vi "Set Control Values v2.vi"(6 "class names":string[](array[string]), 8 "error in":errorcluster, 9 "values":dbl[](array[numeric]), 11 "refnums in":refnum<vi>[](array[refnum])) -> (0 "error out":errorcluster, 3 "refnums out":refnum<vi>[](array[refnum]))   [LabVIEW 2020]
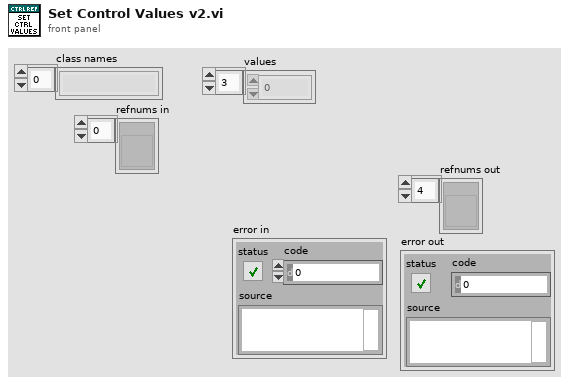
[diagram p1: front panel]
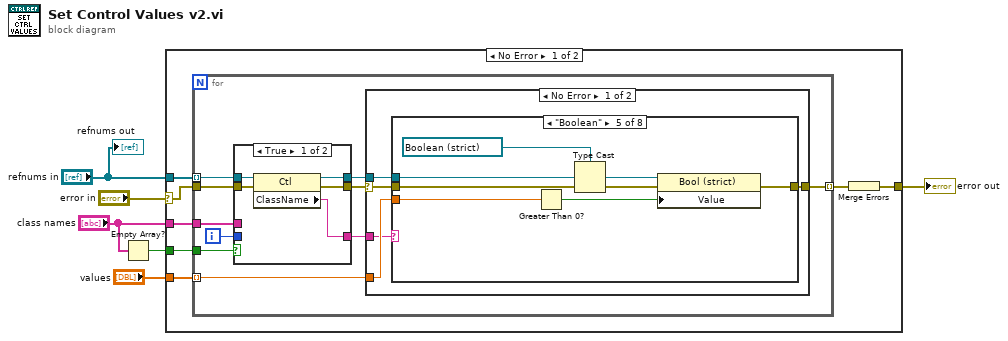
[diagram p0: block diagram]
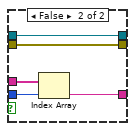
[diagram p2: hidden frame]
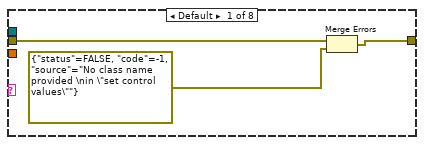
[diagram p3: hidden frame]
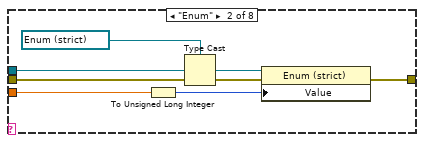
[diagram p4: hidden frame]
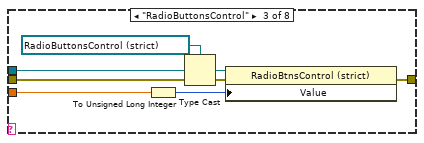
[diagram p5: hidden frame]
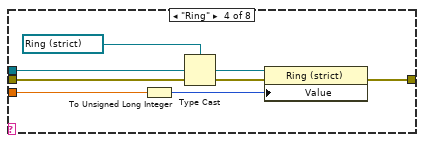
[diagram p6: hidden frame]
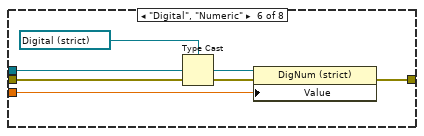
[diagram p7: hidden frame]
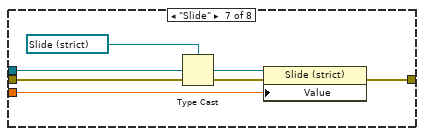
[diagram p8: hidden frame]
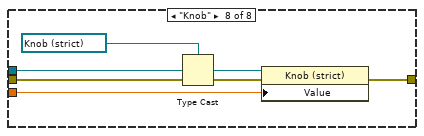
[diagram p9: hidden frame]
diagram:
  n1 = Empty Array?(array="class names") -> (empty?=w3:bool)
  n2 = case shown="No Error" "error in" {
    selector: "error in" -> [w10 w89]
    tunnel: "refnums in" -> [w12 _]
    tunnel: [w11 w89] -> w5
    tunnel: w3 -> [w9 _]
    tunnel: "class names" -> [w8 _]
    tunnel: "values" -> [w7 _]
    frame No Error {
      n3 = for {
        tunnel: w12 -> [w23] mode=indexing
        tunnel: [w21] -> w13 mode=indexing
        tunnel: w10 -> [w19]
        tunnel: w9 -> [w18]
        tunnel: w8 -> [w16]
        tunnel: w7 -> [w14] mode=indexing
        i -> [w15]
        n4 = case shown="True" w18 {
          tunnel: w23 -> [w28 w33]
          tunnel: [w27 w33] -> w22
          tunnel: [w26 w32] -> w20
          tunnel: w19 -> [w25 w32]
          tunnel: [w24 w30] -> w17
          tunnel: w16 -> [_ w31]
          tunnel: w15 -> [_ w29]
          frame True {
            n5 = property class="Ctl"(reference=w28, error in=w25) -> (reference out=w27:refnum<vi>, error out=w26:errorcluster, "ClassName"=w24:string)
          }
          frame False {
            n6 = Index Array(array=w31, index=w29) -> (element=w30:string)
          }
        }
        n7 = case shown="No Error" w20 {
          selector: w20 -> [w38 w88]
          tunnel: w22 -> [w37 _]
          tunnel: [w34 w88] -> w21
          tunnel: w17 -> [w35 _]
          tunnel: w14 -> [w36 _]
          frame No Error {
            n8 = case shown="\"Boolean\"" w35 {
              tunnel: w38 -> [w41 w45 w53 w59 w67 w73 w79 w85]
              tunnel: w37 -> [_ w48 w55 w62 w69 w75 w81 w87]
              tunnel: w36 -> [_ w46 w54 w60 w65 w71 w77 w83]
              tunnel: [w40 w44 w52 w58 w66 w72 w78 w84] -> w34
              frame Default {
                n9 = Merge Errors(w41, errorcluster {"status"=FALSE, "code"=-1, "source"="No class name provided \nin \"set control values\""} ("error constant")) -> (w40:errorcluster)
              }
              frame "Enum" {
                n10 = To Unsigned Long Integer(number=w46) -> (unsigned 32bit integer=w42:u32)
                n11 = Type Cast(type=refnum<vi> refnum ("reference out"), x=w48) -> (*(type *) &x=w47:refnum<vi>)
                n12 = property on="Property Node" class="Enum (strict)"(reference=w47, error in=w45, "Value"=w42) -> (error out=w44:errorcluster)  [unwired: 1 out]
              }
              frame "RadioButtonsControl" {
                n13 = To Unsigned Long Integer(number=w54) -> (unsigned 32bit integer=w51:u32)
                n14 = Type Cast(type=refnum<vi> refnum ("Cooling Mode"), x=w55) -> (*(type *) &x=w49:refnum<vi>)
                n15 = property on="Property Node" class="RadioBtnsControl (strict)"(reference=w49, error in=w53, "Value"=w51) -> (error out=w52:errorcluster)  [unwired: 1 out]
              }
              frame "Ring" {
                n16 = To Unsigned Long Integer(number=w60) -> (unsigned 32bit integer=w56:u32)
                n17 = Type Cast(type=refnum<vi> refnum ("Ring"), x=w62) -> (*(type *) &x=w61:refnum<vi>)
                n18 = property on="Property Node" class="Ring (strict)"(reference=w61, error in=w59, "Value"=w56) -> (error out=w58:errorcluster)  [unwired: 1 out]
              }
              frame "Boolean" {
                n19 = Greater Than 0?(x=w65) -> (x > 0?=w63:bool)
                n20 = Type Cast(type=refnum<vi> refnum ("reference out"), x=w69) -> (*(type *) &x=w68:refnum<vi>)
                n21 = property on="Property Node" class="Bool (strict)"(reference=w68, error in=w67, "Value"=w63) -> (error out=w66:errorcluster)  [unwired: 1 out]
              }
              frame "Digital", "Numeric" {
                n22 = Type Cast(type=refnum<vi> refnum ("reference out"), x=w75) -> (*(type *) &x=w74:refnum<vi>)
                n23 = property on="Property Node" class="DigNum (strict)"(reference=w74, error in=w73, "Value"=w71) -> (error out=w72:errorcluster)  [unwired: 1 out]
              }
              frame "Slide" {
                n24 = Type Cast(type=refnum<vi> refnum ("Slide"), x=w81) -> (*(type *) &x=w80:refnum<vi>)
                n25 = property on="Property Node" class="Slide (strict)"(reference=w80, error in=w79, "Value"=w77) -> (error out=w78:errorcluster)  [unwired: 1 out]
              }
              frame "Knob" {
                n26 = Type Cast(type=refnum<vi> refnum ("Knob"), x=w87) -> (*(type *) &x=w86:refnum<vi>)
                n27 = property on="Property Node" class="Knob (strict)"(reference=w86, error in=w85, "Value"=w83) -> (error out=w84:errorcluster)  [unwired: 1 out]
              }
            }
          }
          frame Error {
          }
        }
      }
      n28 = Merge Errors(w13) -> (w11:errorcluster)
    }
    frame Error {
    }
  }
  "error out" <- w5
  "refnums out" <- "refnums in"
